vi "AttackPsSkill.vi"(9 "Game in":refnum<class "Game.lvclass">, 10 "Robot":refnum<class "Robot.lvclass">, 11 "AttackPsSkill in":refnum<class "AttackPsSkill.lvclass">) -> (2 "Robot out":refnum<class "Robot.lvclass">, 3 "AttackPsSkill out":refnum<class "AttackPsSkill.lvclass">)   [LabVIEW 2023, in "AttackPsSkill.lvclass"]
uses:
  AttackPsSkill.lvclass
  Robot_class/Robot.lvclass
  Game_class/Game.lvclass
panel:
  out "error out 2":errorcluster
  in  "error in (no error) 2":errorcluster
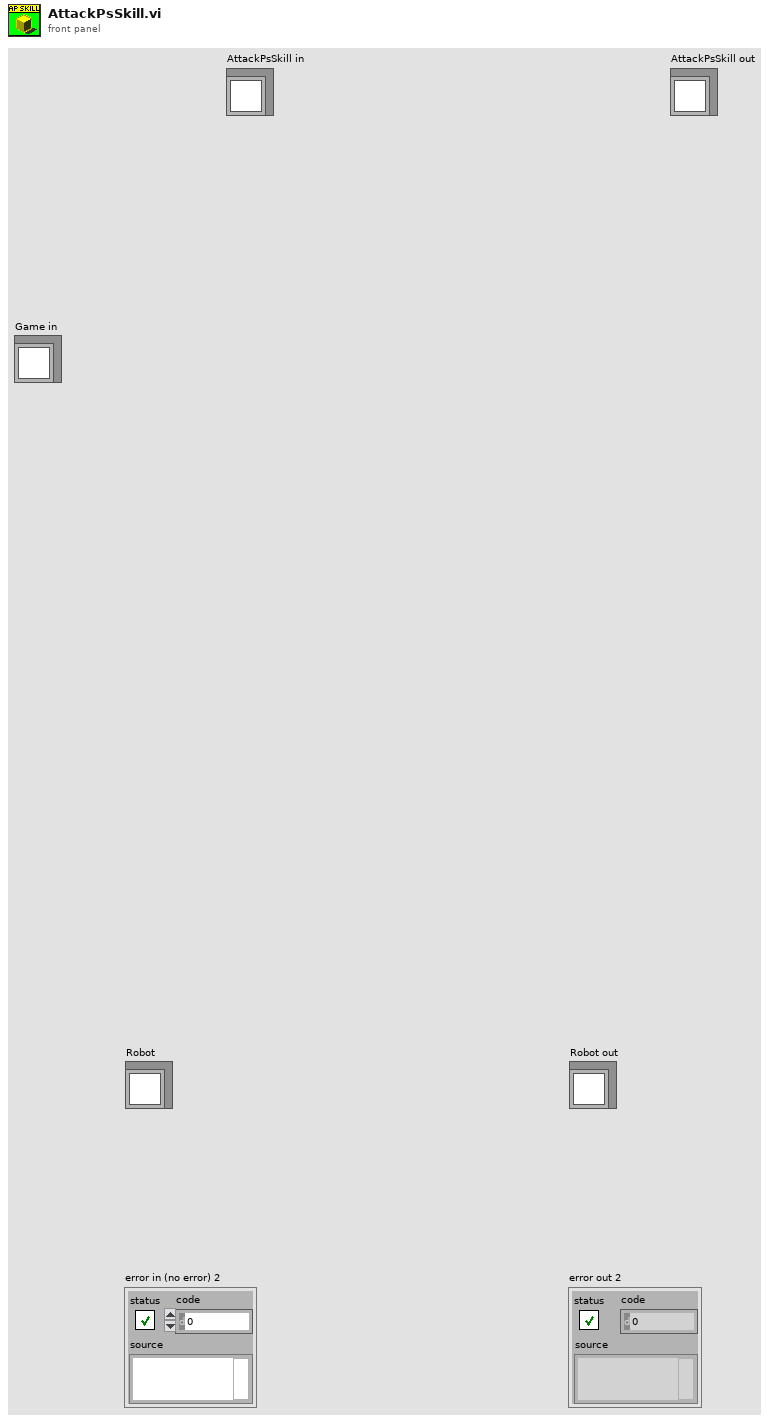
[diagram p1: front panel]
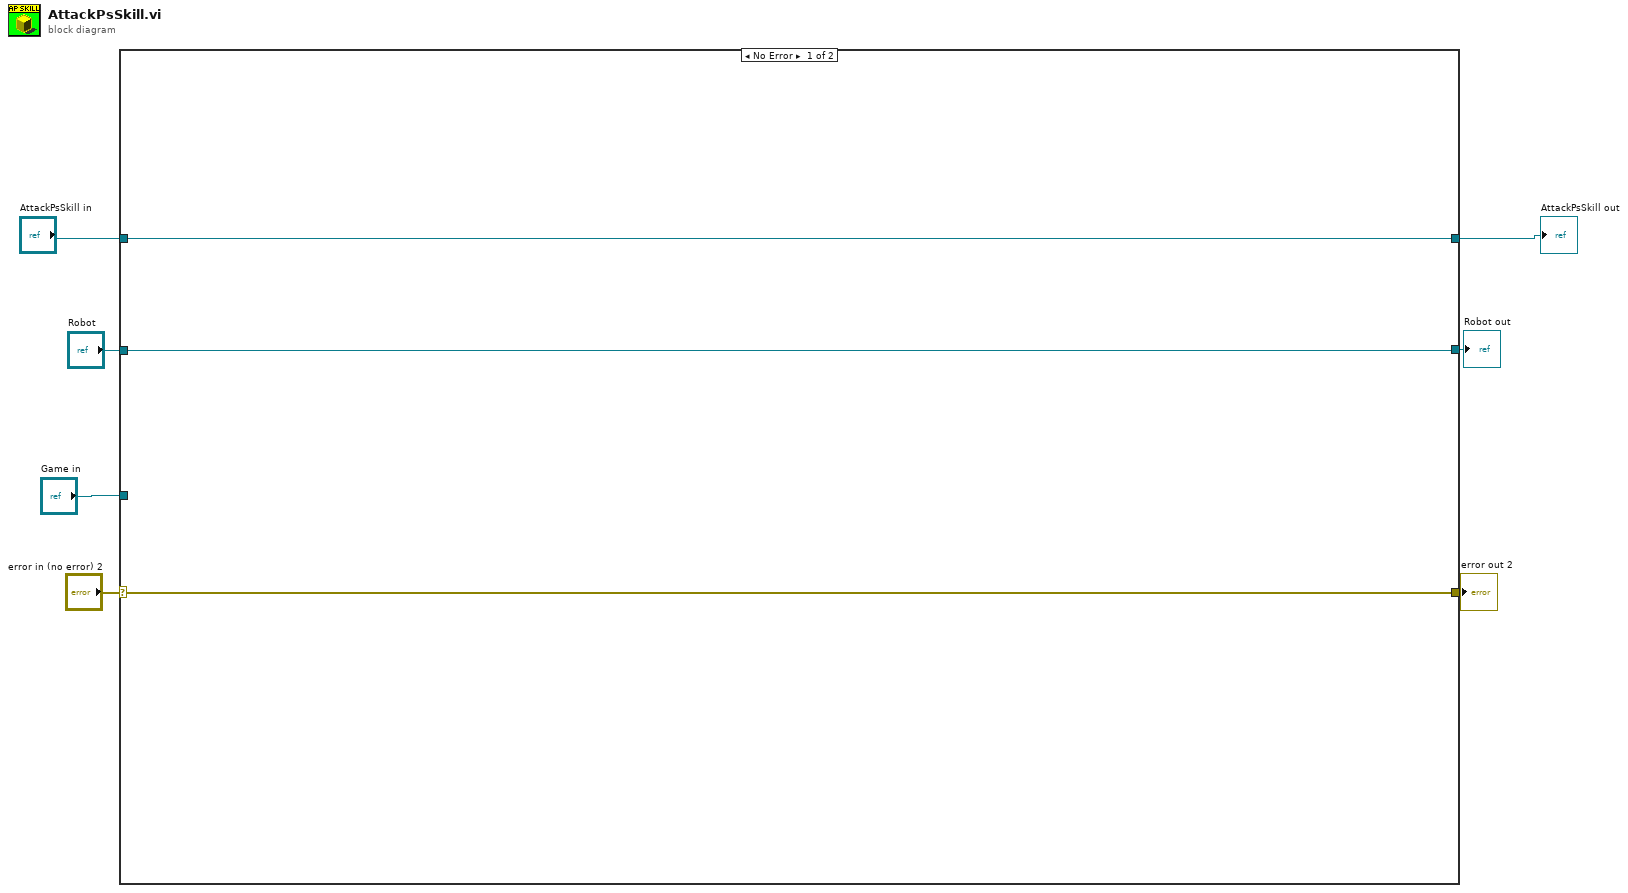
[diagram p0: block diagram]
diagram:
  n1 = case shown="No Error" "error in (no error) 2" {
    selector: "error in (no error) 2" -> [w9 w13]
    tunnel: [w9 w13] -> w6
    tunnel: [w8 w12] -> w3
    tunnel: "AttackPsSkill in" -> [w8 w12]
    tunnel: "Robot" -> [w10 w11]
    tunnel: [w10 w11] -> w4
    tunnel: "Game in" -> [_ _]
    frame No Error {
    }
    frame Error {
    }
  }
  "AttackPsSkill out" <- w3
  "error out 2" <- w6
  "Robot out" <- w4
